vi "FGV-GEvt Filter Rules.vi"(6 "Set? (T)/Get(F)":bool, 8 "Error In":errorcluster caption="error in (no error)", 11 "Rules-v1":T1) -> (0 "error out":errorcluster, 3 "Rules-v1":T1)   [LabVIEW 2017, in "Communicable State Machine.lvlib"]
uses:
  Communicable State Machine.lvlib
  Typedef/_CSM_GlobalLog Filter Rules - v1.0.ctl
  Typedef/_CSM_GlobalLog_MSG_TYPE.ctl
  Typedef/_CSM_GlobalLog_STATE_TYPE.ctl
  ChangeFlag/ChangeFlag-Write.vi
  Utility/Random Change Flag.vi
  ChangeFlag/ChangeFlagDB.vi
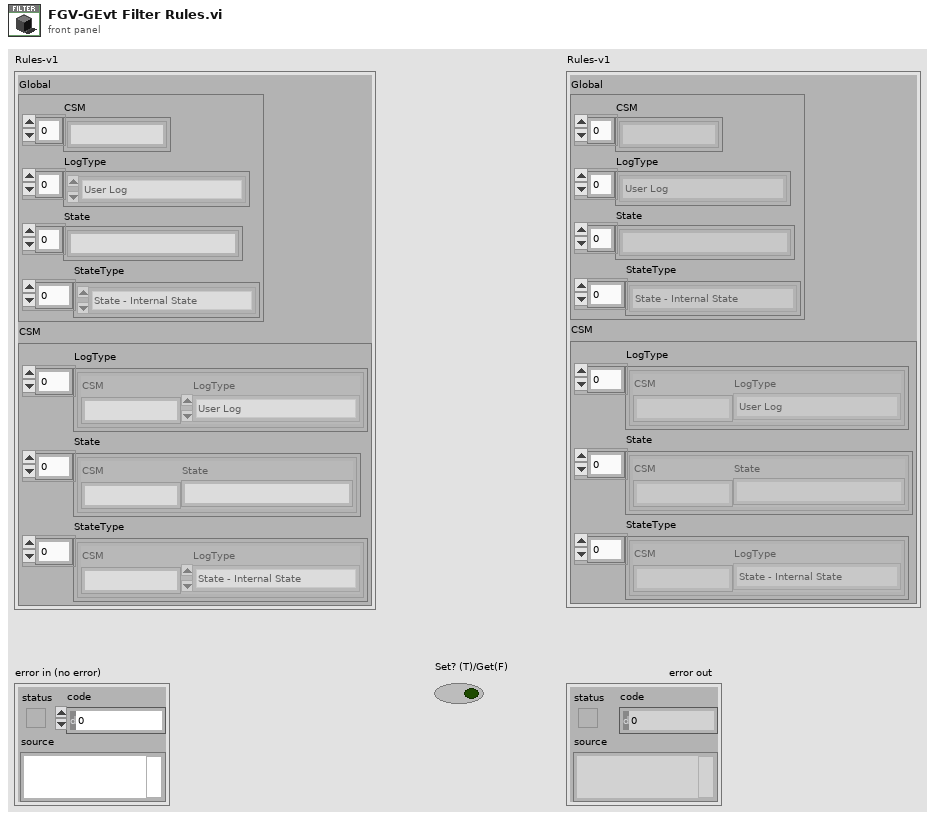
[diagram p1: front panel]
types:
  T1 = typedef "Communicable State Machine.lvlib/_CSM_GlobalLog Filter Rules - v1.0.ctl" = cluster{"Global":cluster{"CSM":string[], "LogType":T2[], "State":string[], "StateType":T3[]}, "CSM":cluster{"LogType":cluster{"CSM":string, "LogType":T2}[], "State":cluster{"CSM":string, "State":string}[], "StateType":cluster{"CSM":string, "LogType":T3}[]}}
  T2 = typedef "Communicable State Machine.lvlib/_CSM_GlobalLog_MSG_TYPE.ctl" = enum16{"User Log", "State Change", "Status", "Interrupt", "Register", "Unregister", "Error Log", "Module Created", "Module Destroyed", "Async Message", "No-Rep Async Message", "Sync Message"}
  T3 = typedef "Communicable State Machine.lvlib/_CSM_GlobalLog_STATE_TYPE.ctl" = enum16{"State - Internal State", "State - External Message", "State - Response", "State - Complete"}
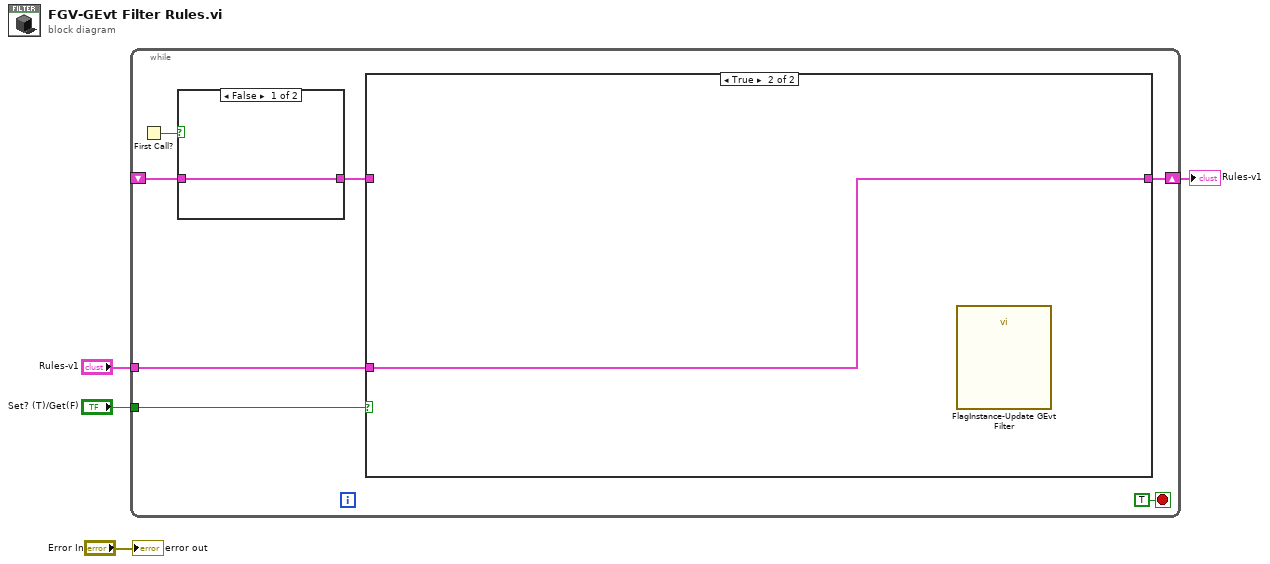
[diagram p0: block diagram]
diagram:
  n1 = while {
    shift-right: [w8] -> w3
    shift-left: _ -> [w7]
    tunnel: "Set? (T)/Get(F)" -> [w6]
    tunnel: "Rules-v1" -> [w5]
    stop <- TRUE stop-if-true
    n2 = First Call?() -> (First Call?: T/F=w10:bool)
    n3 = case shown="False" w10 {
      tunnel: [w12 _] -> w9
      tunnel: w7 -> [w12 _]
      frame False {
      }
      frame True {
      }
    }
    n4 = case shown="True" w6 {
      tunnel: w9 -> [w13 _]
      tunnel: [w13 w14] -> w8
      tunnel: w5 -> [_ w14]
      frame False {
      }
      frame True {
        n5 = call "FlagInstance-Update GEvt Filter.vi"() -> ()  [unwired: 10 in, 2 out]
      }
    }
  }
  "Rules-v1" <- w3
  "error out" <- "Error In"
